vi "PH_SHS_Analysis_Statistician.indicate Result.vi"(0 "i ref in":refnum<vi>, 5 "error in (no error)":errorcluster) -> (14 "i ref out":refnum<vi>, 19 "error out":errorcluster)   [LabVIEW 2014, in "PH_SHS_Analysis_Statistician.lvlib"]
doc: "This VI displays the results"
uses:
  PH_SHS_Analysis_Statistician.lvlib
  <vilib>/Analysis/NI_AALBase.lvlib
  <vilib>/Analysis/NI_AALPro.lvlib
  <vilib>/ptbypt/NI_PtbyPt.lvlib
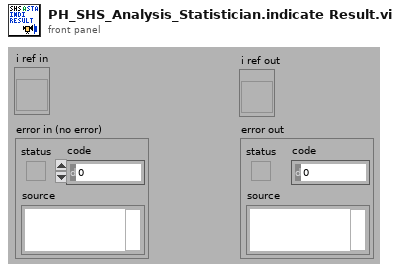
[diagram p1: front panel]
types:
  T1 = typedef "PH_SHS_Analysis_Statistician.lvlib/PH_SHS_Analysis_Statistician.i attribute.ctl" = cluster{"GUI Refs ":cluster{"Status":refnum<vi>, "Result Graph":refnum<vi>, "Mean Data 1":refnum<vi>, "Std Dev Data 1":refnum<vi>, "Mean Data 2":refnum<vi>, "Std Dev Data 2":refnum<vi>, "Mean Data 3":refnum<vi>, "Std Dev Data 3":refnum<vi>, "Dummy Mean":refnum<vi>, "Dummy Std Dev":refnum<vi>, "Export Data":refnum<vi>, "Data 1":refnum<vi>, "Data 2":refnum<vi>, "Data 3":refnum<vi>, "Stat or Trend":refnum<vi>, "Delete":refnum<vi>, "Analyzer":refnum<vi>, "Current Zernike Coefficients":refnum<vi>, "PtV [Lambda]":refnum<vi>, "sample length":refnum<vi>}, "Analyzer":string, "Stat or Trend":bool, "Data 1":i16, "Data 2":i16, "Data 3":i16, "Data":T2[], "sample length":i32, "Datasets strored":i32, "Dataarray Size":i32}
  T2 = typedef "PH_SHS_Analysis.lvlib/PH_SHS_Analysis.Zernike Dataset.ctl" = cluster{"State":T3, "Time Stamp":timestamp, "PtV [lambda]":dbl, "Zernicke Coefficients":T4}
  T3 = typedef "PH_StatusHandler.lvlib/PH_StatusHandler.Status.ctl" = i16
  T4 = typedef "PH_SHS_Analysis.lvlib/PH_SHS_Analysis.Zernike Coefficients.ctl" = cluster{"Tilt x":dbl, "Tilt y":dbl, "Defocus":dbl, "Astig 0°":dbl, "Astig 45°":dbl, "Coma x":dbl, "Coma y":dbl, "Spherical":dbl, "Trefoil 0°":dbl, "Trefoil 30°":dbl, "2nd Astig 0°":dbl, "2nd Astig 45°":dbl, "2nd Coma x":dbl, "2nd Coma y":dbl, "2nd Spherical":dbl}
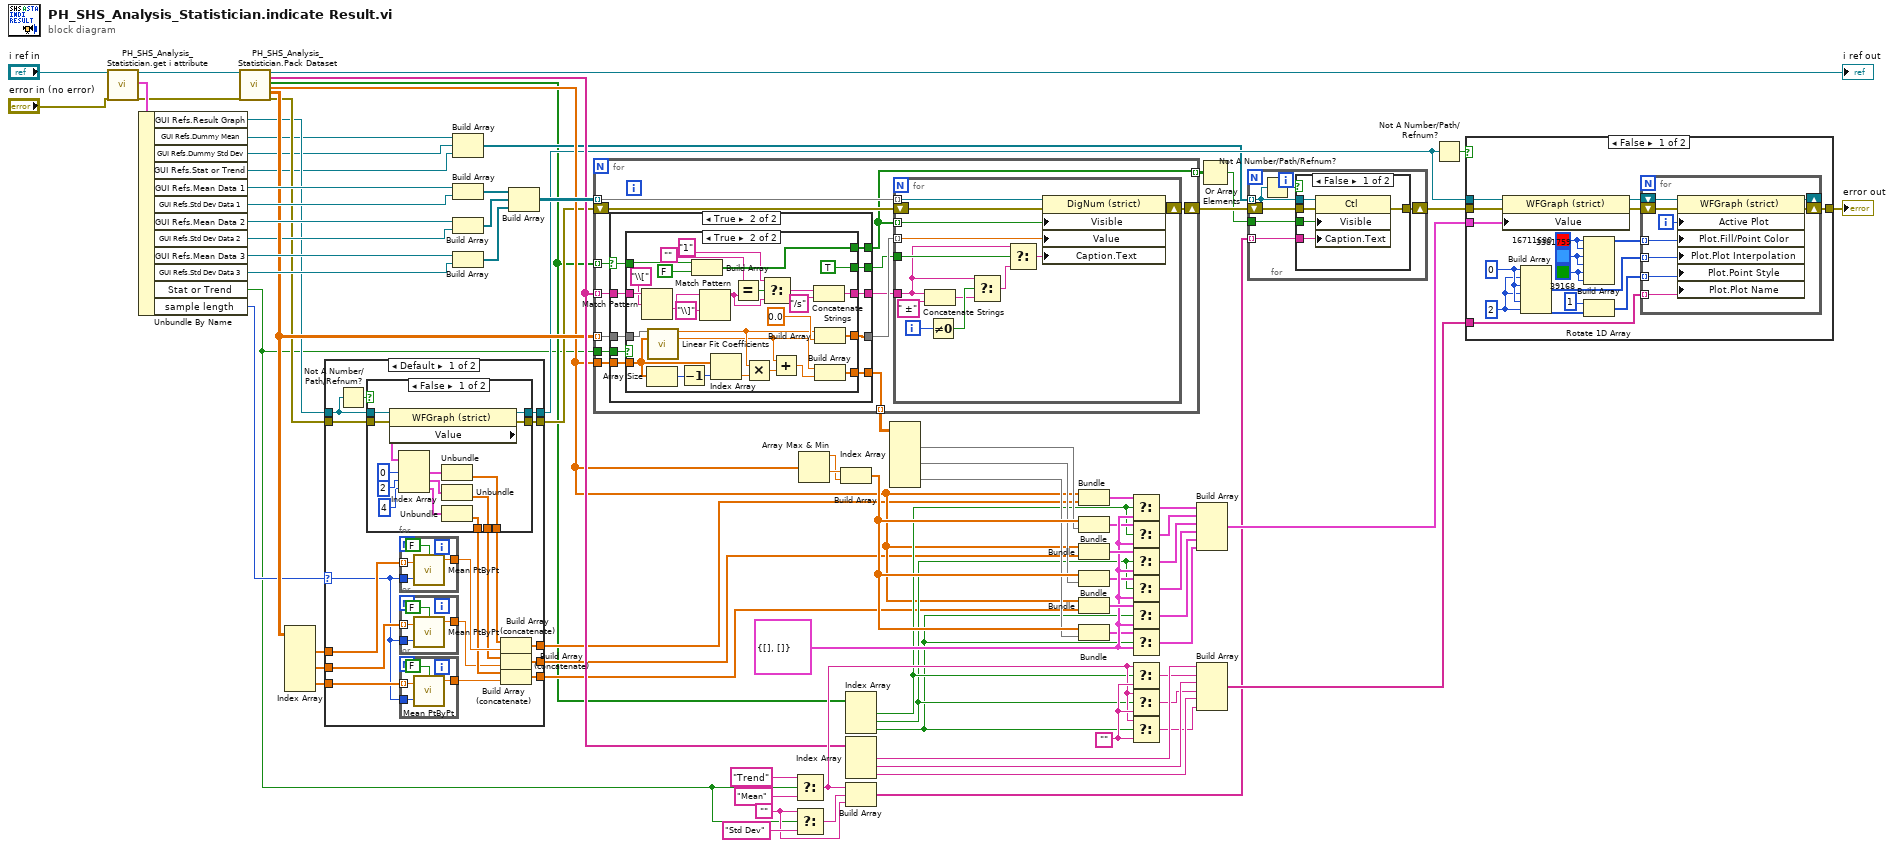
[diagram p0: block diagram]
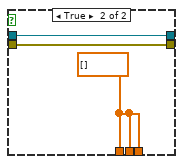
[diagram p3: hidden frame]
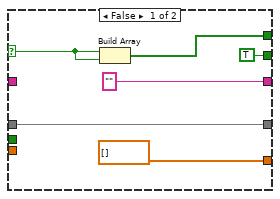
[diagram p6: hidden frame]
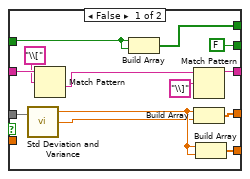
[diagram p7: hidden frame]
diagram:
  w43 = ""
  w50 = ""
  w60 = cluster{dbl[], dbl[]} {[], []} ("output cluster")
  n1 = call "PH_SHS_Analysis_Statistician.get i attribute.vi"("i ref in"="i ref in", "error in (no error)"="error in (no error)") -> ("i ref out"=w26:refnum<vi>, "i attribute"=w79:T1, "error out"=w5:errorcluster)  [unwired: 15 in]
  n2 = Unbundle By Name(w79) -> ("GUI Refs.Result Graph"=w14:refnum<vi>, "GUI Refs.Dummy Mean"=w10:refnum<vi>, "GUI Refs.Dummy Std Dev"=w9:refnum<vi>, "GUI Refs.Stat or Trend"=w8:refnum<vi>, "GUI Refs.Mean Data 1"=w70:refnum<vi>, "GUI Refs.Std Dev Data 1"=w69:refnum<vi>, "GUI Refs.Mean Data 2"=w68:refnum<vi>, "GUI Refs.Std Dev Data 2"=w24:refnum<vi>, "GUI Refs.Mean Data 3"=w71:refnum<vi>, "GUI Refs.Std Dev Data 3"=w72:refnum<vi>, "Stat or Trend"=w1:bool, "sample length"=w17:i32)
  n3 = call "PH_SHS_Analysis_Statistician.Pack Dataset.vi"("i ref in"=w26, "error in"=w5) -> ("i ref out"=→"i ref out":refnum<vi>, "Dataset Legend"=w29:string[], "Dataset chosen?"=w2:bool[], "Timebase"=w27:dbl[], "Dataset"=w28:dbl[][], "error out"=w16:errorcluster)  [unwired: 12 in]
  n4 = Index Array(array=w28) -> (element #1=w23:dbl[], element #2=w21:dbl[], element #3=w19:dbl[])  [unwired: 6 in]
  n5 = case shown="Default" w17 {
    selector: w17 -> [w96 _]
    tunnel: w23 -> [w99 w133]
    tunnel: [w85 w133] -> w22
    tunnel: w21 -> [w97 w132]
    tunnel: [w86 w132] -> w20
    tunnel: w19 -> [w98 w131]
    tunnel: [w87 w131] -> w18
    tunnel: w16 -> [w95 w130]
    tunnel: [w94 w130] -> w15
    tunnel: w14 -> [w92 w129]
    tunnel: [w82 w129] -> w13
    frame Default {
      n6 = Not A Number/Path/Refnum?(number/path/refnum=w92) -> (NaN/Path/Refnum?=w93:bool)
      n7 = case shown="False" w93 {
        tunnel: w95 -> [w113 w116]
        tunnel: [w112 w116] -> w94
        tunnel: w92 -> [w111 w114]
        tunnel: [w108 w115] -> w91
        tunnel: [w105 w115] -> w89
        tunnel: [w104 w115] -> w88
        tunnel: [w103 w114] -> w82
        frame False {
          n8 = property class="WFGraph (strict)"(reference=w111, error in=w113) -> (reference out=w103:refnum<vi>, error out=w112:errorcluster, "Value"=w110:cluster{dbl[], dbl[]}[])
          n9 = Index Array(array=w110, index #1=0 ("index"), index #2=2 ("index"), index #3=4 ("index")) -> (element #1=w109:cluster{dbl[], dbl[]}, element #2=w107:cluster{dbl[], dbl[]}, element #3=w106:cluster{dbl[], dbl[]})
          n10 = Unbundle(w109) -> (w108:dbl[])  [unwired: 1 out]
          n11 = Unbundle(w107) -> (w105:dbl[])  [unwired: 1 out]
          n12 = Unbundle(w106) -> (w104:dbl[])  [unwired: 1 out]
        }
        frame True {
          w115 = dbl[] []
        }
      }
      n13 = for {
        tunnel: w99 -> [w128] mode=indexing
        tunnel: w96 -> [w127]
        tunnel: [w126] -> w90
        n14 = call <vilib>:"Mean PtByPt.vi"("x"=w128, "sample length"=w127, "initialize"=FALSE) -> ("mean"=w126:dbl)  [unwired: 1 in, 1 out]
      }
      n15 = for {
        tunnel: w97 -> [w124] mode=indexing
        tunnel: w96 -> [w123]
        tunnel: [w122] -> w83
        n16 = call <vilib>:"Mean PtByPt.vi"("x"=w124, "sample length"=w123, "initialize"=FALSE) -> ("mean"=w122:dbl)  [unwired: 1 in, 1 out]
      }
      n17 = for {
        tunnel: w98 -> [w120] mode=indexing
        tunnel: w96 -> [w119]
        tunnel: [w118] -> w84
        n18 = call <vilib>:"Mean PtByPt.vi"("x"=w120, "sample length"=w119, "initialize"=FALSE) -> ("mean"=w118:dbl)  [unwired: 1 in, 1 out]
      }
      n19 = Build Array (concatenate)(w91, w90) -> (w85:dbl[])
      n20 = Build Array (concatenate)(w89, w83) -> (w86:dbl[])
      n21 = Build Array (concatenate)(w88, w84) -> (w87:dbl[])
    }
    frame 1 {
    }
  }
  n22 = Build Array(w10, w9, w8) -> (w7:refnum<vi>[])
  n23 = Build Array(w70, w69) -> (w67:refnum<vi>[])
  n24 = Build Array(w68, w24) -> (w66:refnum<vi>[])
  n25 = Build Array(w71, w72) -> (w65:refnum<vi>[])
  n26 = Build Array(w67, w66, w65) -> (w49:refnum<vi>[][])
  n27 = for {
    tunnel: w28 -> [w146] mode=indexing
    tunnel: w49 -> [w145] mode=indexing
    shift-right: [w143] -> w12
    shift-left: w15 -> [w142]
    tunnel: w2 -> [w139] mode=indexing
    tunnel: w29 -> [w141] mode=indexing
    tunnel: [w137] -> w61 mode=indexing
    tunnel: w1 -> [w138]
    tunnel: w27 -> [w136]
    tunnel: [w134] -> w4 mode=indexing
    n28 = case shown="True" w139 {
      selector: w139 -> [w150 w158]
      tunnel: w146 -> [w151 w162]
      tunnel: [w151 w161] -> w144
      tunnel: w141 -> [_ w160]
      tunnel: ["" ("Data Legend") w159] -> w140
      tunnel: [w149 w157] -> w134
      tunnel: w138 -> [_ w156]
      tunnel: [dbl[] [] w155] -> w137
      tunnel: w136 -> [_ w154]
      tunnel: [TRUE w153] -> w135
      frame False {
        n29 = Build Array(w150, w150) -> (w149:bool[])
      }
      frame True {
        n30 = case shown="True" w156 {
          tunnel: w162 -> [w166 w186]
          tunnel: [w175 w202] -> w161
          tunnel: w160 -> [w174 w201]
          tunnel: [w170 w188] -> w159
          tunnel: w158 -> [w169 w197]
          tunnel: [w168 w196] -> w157
          tunnel: [w167 w185] -> w155
          tunnel: w154 -> [_ w184]
          tunnel: [FALSE TRUE] -> w153
          frame False {
            n31 = call <vilib>:"Std Deviation and Variance.vi"("X"=w166) -> ("mean"=w165:dbl, "standard deviation"=w164:dbl)  [unwired: 1 in, 1 out]
            n32 = Match Pattern(string=w174, regular expression="\\[") -> (after substring=w172:string)  [unwired: 1 in, 3 out]
            n33 = Build Array(w169, w169) -> (w168:bool[])
            n34 = Match Pattern(string=w172, regular expression="\\]") -> (before substring=w170:string)  [unwired: 1 in, 3 out]
            n35 = Build Array(w165, w164) -> (w175:dbl[])
            n36 = Build Array(w165, w165) -> (w167:dbl[])
          }
          frame True {
            n37 = Match Pattern(string=w201, regular expression="\\[") -> (after substring=w199:string)  [unwired: 1 in, 3 out]
            n38 = Array Size(array=w184) -> (size(s)=w183:i32)
            n39 = call <vilib>:"Linear Fit Coefficients.vi"("Y"=w186, "X"=w184) -> ("slope"=w180:dbl, "intercept"=w178:dbl)  [unwired: 11 in, 1 out]
            n40 = Decrement(x=w183) -> (x-1=w182:i32)
            n41 = Build Array(w197, FALSE ("element")) -> (w196:bool[])
            n42 = Match Pattern(string=w199, regular expression="\\]") -> (before substring=w191:string)  [unwired: 1 in, 3 out]
            n43 = Index Array(array=w184, index=w182) -> (element=w181:dbl)
            n44 = Equal?(x="", y=w191) -> (x = y?=w192:bool)
            n45 = Multiply(x=w180, y=w181) -> (x*y=w179:dbl)
            n46 = Select(t="1" ("regular expression"), s=w192, f=w191) -> (s? t:f=w189:string)
            n47 = Add(x=w178, y=w179) -> (x+y=w177:dbl)
            n48 = Concatenate Strings(w189, "/s" ("regular expression")) -> (w188:string)
            n49 = Build Array(w180, 0.0 ("element")) -> (w202:dbl[])
            n50 = Build Array(w178, w177) -> (w185:dbl[])
          }
        }
      }
    }
    n51 = for {
      tunnel: w145 -> [w215] mode=indexing
      tunnel: w144 -> [w214] mode=indexing
      shift-right: [w212] -> w143
      shift-left: w142 -> [w213]
      tunnel: w134 -> [w211] mode=indexing
      tunnel: w140 -> [w203]
      tunnel: w135 -> [w204]
      i -> [w206]
      n52 = Concatenate Strings(w203, " ±") -> (w208:string)
      n53 = Not Equal To 0?(x=w206) -> (x != 0?=w210:bool)
      n54 = Select(t=w203, s=w210, f=w208) -> (s? t:f=w207:string)
      n55 = Select(t=w203, s=w204, f=w207) -> (s? t:f=w205:string)
      n56 = property class="DigNum (strict)"(reference=w215, error in=w213, "Visible"=w211, "Value"=w214, "Caption.Text"=w205) -> (error out=w212:errorcluster)  [unwired: 1 out]
    }
  }
  n57 = Select(t="Trend" ("Plot.Plot Name"), s=w1, f="Mean") -> (s? t:f=w44:string)
  n58 = Select(t=w43, s=w1, f="Std Dev") -> (s? t:f=w48:string)
  n59 = Array Max & Min(array=w27) -> (max value=w63:dbl, min value=w64:dbl)  [unwired: 2 out]
  n60 = Build Array(w64, w63) -> (w62:dbl[])
  n61 = Index Array(array=w2) -> (element #1=w34:bool, element #2=w33:bool, element #3=w32:bool)  [unwired: 3 in]
  n62 = Index Array(array=w29) -> (element #1=w42:string, element #2=w41:string, element #3=w40:string)  [unwired: 3 in]
  n63 = Build Array(w44, w48, w43) -> (w6:string[])
  n64 = Index Array(array=w61) -> (element #1=w53:dbl[], element #2=w52:dbl[], element #3=w51:dbl[])  [unwired: 6 in]
  n65 = Bundle("Timebase"=w27, "Dataset"=w22) -> (w78:cluster{"Timebase":dbl[], "Dataset":dbl[]})  [unwired: 1 in]
  n66 = Bundle(w62, w53) -> (w57:cluster{dbl[], dbl[]})  [unwired: 1 in]
  n67 = Bundle("Timebase"=w27, "Dataset"=w20) -> (w76:cluster{"Timebase":dbl[], "Dataset":dbl[]})  [unwired: 1 in]
  n68 = Bundle(w62, w52) -> (w58:cluster{dbl[], dbl[]})  [unwired: 1 in]
  n69 = Bundle("Timebase"=w27, "Dataset"=w18) -> (w75:cluster{"Timebase":dbl[], "Dataset":dbl[]})  [unwired: 1 in]
  n70 = Bundle(w62, w51) -> (w59:cluster{dbl[], dbl[]})  [unwired: 1 in]
  n71 = Select(t=w78, s=w34, f=w60) -> (s? t:f=w77:cluster{"Timebase":dbl[], "Dataset":dbl[]})
  n72 = Select(t=w57, s=w34, f=w60) -> (s? t:f=w56:cluster{dbl[], dbl[]})
  n73 = Select(t=w76, s=w33, f=w60) -> (s? t:f=w74:cluster{"Timebase":dbl[], "Dataset":dbl[]})
  n74 = Select(t=w58, s=w33, f=w60) -> (s? t:f=w55:cluster{dbl[], dbl[]})
  n75 = Select(t=w75, s=w32, f=w60) -> (s? t:f=w73:cluster{"Timebase":dbl[], "Dataset":dbl[]})
  n76 = Select(t=w59, s=w32, f=w60) -> (s? t:f=w54:cluster{dbl[], dbl[]})
  n77 = Select(t=w44, s=w34, f=w50) -> (s? t:f=w39:string)
  n78 = Select(t=w44, s=w33, f=w50) -> (s? t:f=w38:string)
  n79 = Select(t=w44, s=w32, f=w50) -> (s? t:f=w37:string)
  n80 = Build Array(w77, w56, w74, w55, w73, w54) -> (w35:cluster{"Timebase":dbl[], "Dataset":dbl[]}[])
  n81 = Build Array(w42, w39, w41, w38, w40, w37) -> (w36:string[])
  n82 = Or Array Elements(Boolean array=w4) -> (logical OR=w3:bool)
  n83 = for {
    tunnel: w7 -> [w217] mode=indexing
    shift-right: [w220] -> w11
    shift-left: w12 -> [w221]
    tunnel: w6 -> [w219] mode=indexing
    tunnel: w3 -> [w216]
    n84 = Not A Number/Path/Refnum?(number/path/refnum=w217) -> (NaN/Path/Refnum?=w218:bool)
    n85 = case shown="False" w218 {
      tunnel: w217 -> [w226 _]
      tunnel: w221 -> [w225 w227]
      tunnel: [w224 w227] -> w220
      tunnel: w219 -> [w223 _]
      tunnel: w216 -> [w222 _]
      frame False {
        n86 = property class="Ctl"(reference=w226, error in=w225, "Visible"=w222, "Caption.Text"=w223) -> (error out=w224:errorcluster)  [unwired: 1 out]
      }
      frame True {
      }
    }
  }
  n87 = Not A Number/Path/Refnum?(number/path/refnum=w13) -> (NaN/Path/Refnum?=w30:bool)
  n88 = case shown="False" w30 {
    tunnel: w36 -> [w234 _]
    tunnel: w35 -> [w233 _]
    tunnel: w13 -> [w232 _]
    tunnel: w11 -> [w230 w253]
    tunnel: [w228 w253] -> w31
    frame False {
      w238 = u8 2 ("Plot.Plot Interpolation")
      w239 = u8 0 ("Plot.Plot Interpolation")
      w242 = u32 39168 ("Color Box")
      w241 = u32 3381759 ("Color Box")
      w243 = u32 16711680 ("Color Box")
      n89 = property class="WFGraph (strict)"(reference=w232, error in=w230, "Value"=w233) -> (reference out=w231:refnum<vi>, error out=w229:errorcluster)
      n90 = Build Array(w239, w238, w239, w238, w239, w238) -> (w237:u8[])
      n91 = Build Array(w243, w243, w241, w241, w242, w242) -> (w240:u32[])
      n92 = Rotate 1D Array(1:w237, 2:1 ("n")) -> (0:w235:u8[])
      n93 = for {
        shift-right: [w252] -> _
        shift-left: w231 -> [w251]
        shift-right: [w250] -> w228
        shift-left: w229 -> [w249]
        tunnel: w240 -> [w247] mode=indexing
        tunnel: w237 -> [w246] mode=indexing
        tunnel: w235 -> [w245] mode=indexing
        tunnel: w234 -> [w244] mode=indexing
        i -> [w248]
        n94 = property class="WFGraph (strict)"(reference=w251, error in=w249, "Active Plot"=w248, "Plot.Fill/Point Color"=w247, "Plot.Plot Interpolation"=w246, "Plot.Point Style"=w245, "Plot.Plot Name"=w244) -> (reference out=w252:refnum<vi>, error out=w250:errorcluster)
      }
    }
    frame True {
    }
  }
  "error out" <- w31
